vi "CRYStimulus Wave.vi"(7 "EQ Curve":T1={"Name"="", "Curve"=[], "X data"=1, "Y data"=1, "Z data"=1, "X axis"=0, "Y axis"=1, "Z axis"=1, "X unit"="Hz", "Y unit"="", "Z unit"="deg.", "X dB ref"=1.0, "Y dB ref"=1.0, "Z dB ref"=1.0, "single val"=FALSE, "protected"=FALSE, "display X"=TRUE, "display Y"=TRUE, "display Z"=TRUE, "Test Info"="", "Step No."=0, "Plot Settings"={"Color"=0, "Interpolation"=0, "Point Style"=0, "Line Style"=0, "Point Color"=0, "Line Width"=0, "Bar Plot Style"=0, "Fill To"=0}, "AutoProtect"=FALSE} {"Z data" items=["dB", "Lin"]; "X data" items=["dB", "Lin"]; "Y data" items=["dB", "Lin"]; "Z dB ref" format="%.1f"; "Z axis" items=["Log", "Lin"]; "X dB ref" format="%.1f"; "X axis" items=["Log", "Lin"]; "Y axis" items=["Log", "Lin"]; "Y dB ref" format="%.1f"; "Curve"."z" format="%.2f"; "Curve"."y" format="%.2f"; "Curve"."x" format="%.2f"}, 8 "Output Flag":cluster{bool, bool, "ApplyEQ":bool}, 9 "Max level":dbl format="%.2f", 10 "Level Out":dbl format="%.2f", 11 "wav path":path) -> (0 "Verdict":bool, 1 "Stop Frequency":dbl=100.0 format="%_4f", 2 "Start Frequency":dbl=1.0, 3 "Sampling Rate":dbl=44100.0 format="%.2f", 4 "R":sgl[](array[numeric]), 5 "Channel":enum16{"Left", "Right", "Neither"}[](array[ring]), 6 "L":sgl[](array[numeric]))   [LabVIEW 2013]
uses:
  Typedef Control/CRYData Cluster.ctl
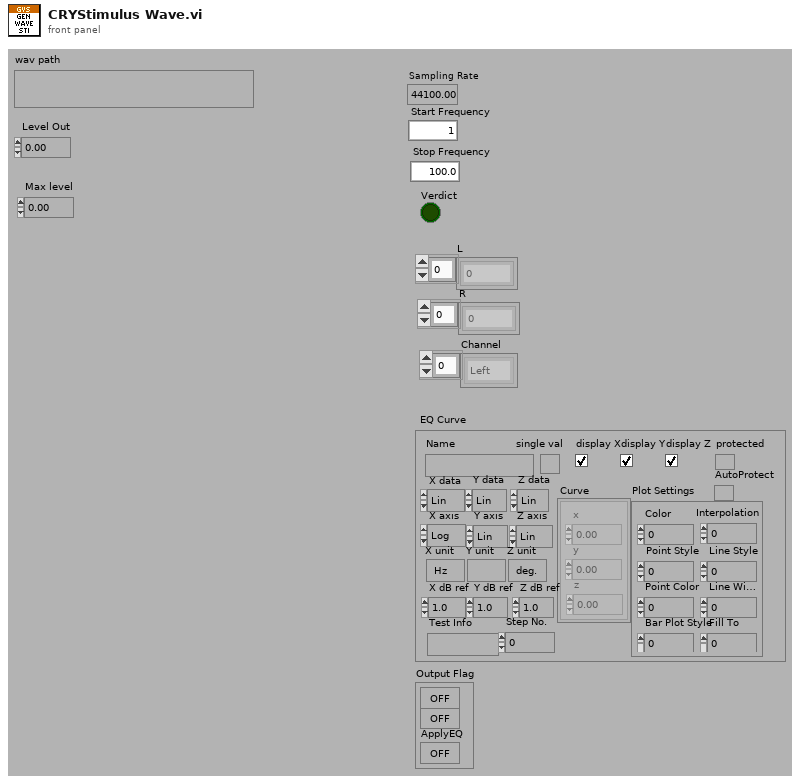
[diagram p1: front panel]
types:
  T1 = typedef "CRYData Cluster.ctl" = cluster{"Name":string, "Curve":cluster{"x":dbl, "y":dbl, "z":dbl}[], "X data":u16, "Y data":u16, "Z data":u16, "X axis":u16, "Y axis":u16, "Z axis":u16, "X unit":string, "Y unit":string, "Z unit":string, "X dB ref":dbl, "Y dB ref":dbl, "Z dB ref":dbl, "single val":bool, "protected":bool, "display X":bool, "display Y":bool, "display Z":bool, "Test Info":string, "Step No.":i32, "Plot Settings":cluster{"Color":u32, "Interpolation":u8, "Point Style":u8, "Line Style":u8, "Point Color":u32, "Line Width":u8, "Bar Plot Style":u8, "Fill To":i16}, "AutoProtect":bool}
  T2 = typedef "Sound Data Format.ctl" = cluster{"sample rate (S/s)":dbl, "number of channels":i32, "bits per sample":i32}
  T3 = typedef "CRYWaveFile Information Typedef.ctl" = cluster{"total number of samples/ch":u32, "total byte number":u32, "Time DBL":dbl, "format str":string, "Time Str":string, "peak FSD":dbl, "rms FSD":dbl, "peak %FSD":dbl, "rms %FSD":dbl, "rms":dbl, "Channel Number":u16, "rms L":dbl, "rms R":dbl}
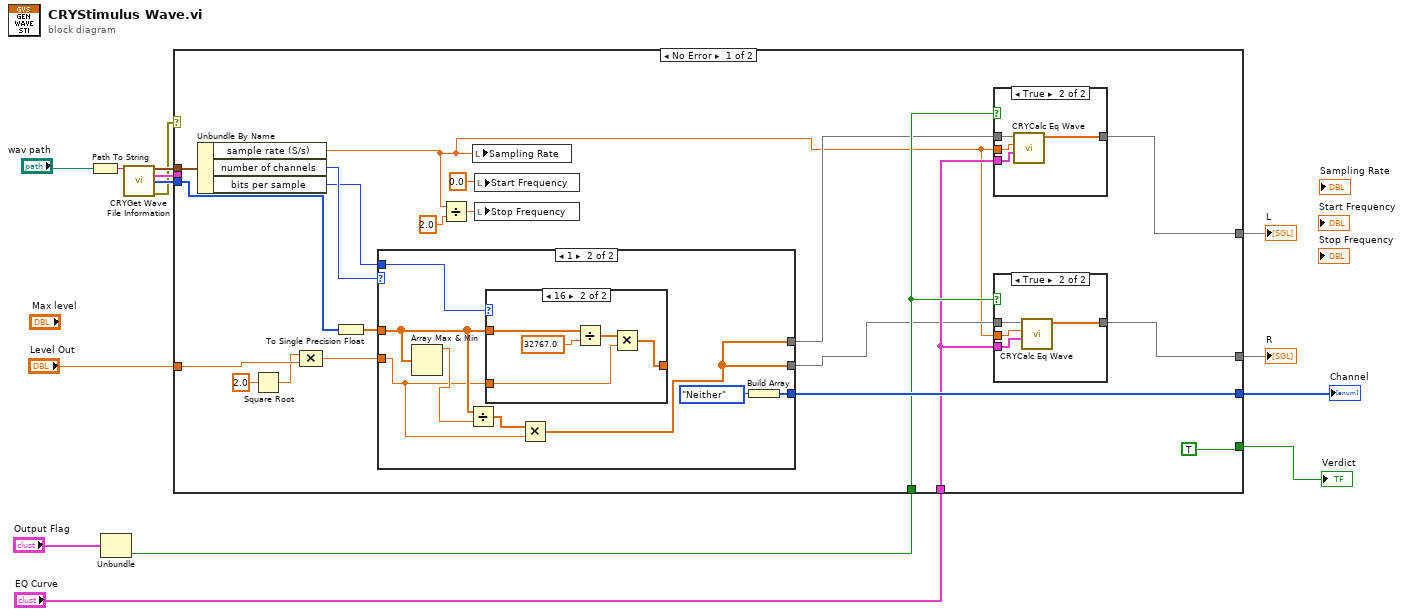
[diagram p0: block diagram]
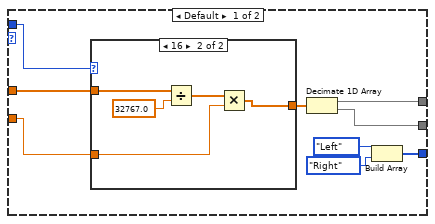
[diagram p4: hidden frame]
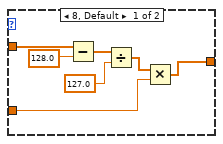
[diagram p5: hidden frame]
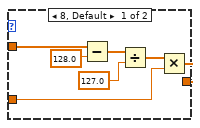
[diagram p6: hidden frame]
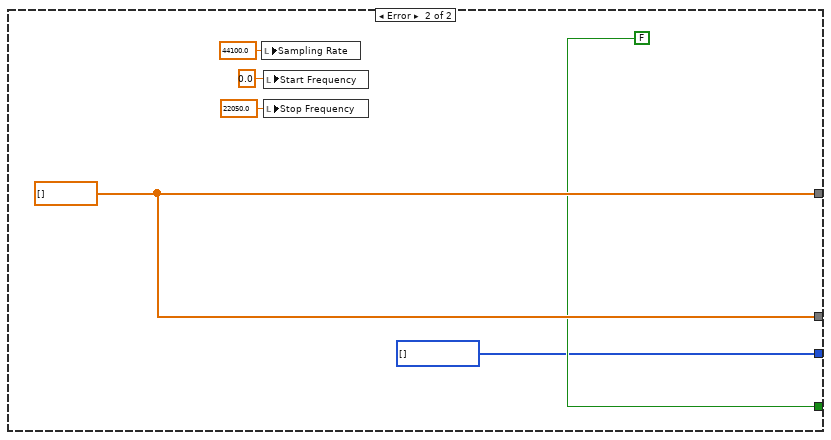
[diagram p7: hidden frame]
diagram:
  n1 = Path To String(path="wav path") -> (string=w13:string)
  n2 = Unbundle("Output Flag") -> ("ApplyEQ"=w2:bool)  [unwired: 2 out]
  n3 = call "CRYGet Wave File Information.vi"("FileNameStr"=w13) -> ("sound format"=w12:T2, "wave info"=w11:T3, "wave data out"=w10:i32[], "Error Output"=w9:errorcluster)  [unwired: 11 out]
  n4 = case shown="No Error" w9 {
    tunnel: [w16 w92] -> w6
    tunnel: [w15 w92] -> w5
    tunnel: "Level Out" -> [w34 _]
    tunnel: [TRUE ("Verdict") FALSE ("Verdict")] -> w7
    tunnel: w12 -> [w28 _]
    tunnel: w11 -> [_ _]
    tunnel: w10 -> [w24 _]
    tunnel: [w22 w87] -> w4
    tunnel: w2 -> [w21 _]
    tunnel: "EQ Curve" -> [w19 _]
    frame No Error {
      n5 = Unbundle By Name(w28) -> ("sample rate (S/s)"=w17:dbl, "number of channels"=w27:i32, "bits per sample"=w25:i32)
      n6 = Square Root(x=2.0) -> (sqrt(x)=w31:dbl)
      n7 = Compound Arithmetic op=MULTIPLY(w31, w34) -> (w26:dbl)
      n8 = To Single Precision Float(number=w24) -> (single precision float=w23:sgl[])
      n9 = case shown="1" w27 {
        tunnel: w23 -> [w52 w70]
        tunnel: [w50 w67] -> w20
        tunnel: [w49 w67] -> w18
        tunnel: w26 -> [w54 w68]
        tunnel: w25 -> [w53 w74]
        tunnel: [w46 w72] -> w22
        frame Default {
          n10 = case shown="16" w53 {
            tunnel: w54 -> [w57 w64]
            tunnel: w52 -> [w56 w65]
            tunnel: [w55 w63] -> w51
            frame 8, Default {
              n11 = Subtract(x=w56, y=128.0) -> (x-y=w60:dbl[])
              n12 = Divide(x=w60, y=127.0) -> (x/y=w61:dbl[])
              n13 = Multiply(x=w61, y=w57) -> (x*y=w55:dbl[])
            }
            frame 16 {
              n14 = Divide(x=w65, y=32767.0) -> (x/y=w66:dbl[])
              n15 = Multiply(x=w66, y=w64) -> (x*y=w63:dbl[])
            }
          }
          n16 = Decimate 1D Array(w51) -> (w50:dbl[], w49:dbl[])
          n17 = Build Array(enum16{"Left", "Right", "Neither"}."Left" ("Enum"), enum16{"Left", "Right", "Neither"}."Right" ("Enum")) -> (w46:enum16{"Left", "Right", "Neither"}[])
        }
        frame 1 {
          n18 = Array Max & Min(array=w70) -> (max value=w71:sgl)  [unwired: 3 out]
          n19 = Divide(x=w70, y=w71) -> (x/y=w69:sgl[])
          n20 = case shown="16" w74 {
            tunnel: w68 -> [w77 w84]
            tunnel: w70 -> [w76 w85]
            tunnel: [w75 w83] -> _
            frame 8, Default {
              n21 = Subtract(x=w76, y=128.0) -> (x-y=w80:dbl[])
              n22 = Divide(x=w80, y=127.0) -> (x/y=w81:dbl[])
              n23 = Multiply(x=w81, y=w77) -> (x*y=w75:dbl[])
            }
            frame 16 {
              n24 = Divide(x=w85, y=32767.0) -> (x/y=w86:dbl[])
              n25 = Multiply(x=w86, y=w84) -> (x*y=w83:dbl[])
            }
          }
          n26 = Multiply(x=w69, y=w68) -> (x*y=w67:dbl[])
          n27 = Build Array(enum16{"Left", "Right", "Neither"}."Neither" ("Enum")) -> (w72:enum16{"Left", "Right", "Neither"}[])
        }
      }
      n28 = Divide(x=w17, y=2.0 ("x")) -> (x/y=w29:dbl)
      n29 = local write "Sampling Rate"(w17) -> ()
      n30 = local write "Start Frequency"(0.0 ("Start Frequency")) -> ()
      n31 = local write "Stop Frequency"(w29) -> ()
      n32 = case shown="True" w21 {
        tunnel: w19 -> [_ w45]
        tunnel: w17 -> [_ w44]
        tunnel: w20 -> [w41 w43]
        tunnel: [w41 w42] -> w16
        frame False {
        }
        frame True {
          n33 = call "CRYCalc Eq Wave.vi"("EQ Curve"=w45, "Fs"=w44, "Wave In"=w43) -> ("Wave Out"=w42:dbl[])  [unwired: 7 in, 1 out]
        }
      }
      n34 = case shown="True" w21 {
        tunnel: w19 -> [_ w40]
        tunnel: w17 -> [_ w39]
        tunnel: w18 -> [w36 w38]
        tunnel: [w36 w37] -> w15
        frame False {
        }
        frame True {
          n35 = call "CRYCalc Eq Wave.vi"("EQ Curve"=w40, "Fs"=w39, "Wave In"=w38) -> ("Wave Out"=w37:dbl[])  [unwired: 7 in, 1 out]
        }
      }
    }
    frame Error {
      w87 = enum16{"Left", "Right", "Neither"}[] [] items=["Left", "Right", "Neither"]
      w92 = sgl[] []
      n36 = local write "Sampling Rate"(44100.0 ("Sampling Rate")) -> ()
      n37 = local write "Start Frequency"(0.0 ("Start Frequency")) -> ()
      n38 = local write "Stop Frequency"(22050.0 ("Stop Frequency")) -> ()
    }
  }
  "Verdict" <- w7
  "L" <- w6
  "R" <- w5
  "Channel" <- w4
